vi "niRFSTS SG Set Waveform Names.vi"(0 "TSM Context in":T1, 5 "Waveform Names":string[](array[string]), 11 "error in (no error)":errorcluster) -> (4 "TSM Context out":T1, 15 "error out":errorcluster)   [LabVIEW 2014]
uses:
  <vilib>/NI_TestStand_SemiconductorModule/NI_TestStand_Semiconductor_Module.lvlibp/PinMap/General/SemiconductorModuleContext.ctl
  <vilib>/NI_TestStand_SemiconductorModule/NI_TestStand_Semiconductor_Module.lvlibp
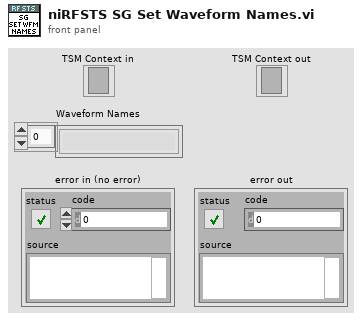
[diagram p1: front panel]
types:
  T1 = typedef "NI_TestStand_Semiconductor_Module.lvlibp/SemiconductorModuleContext.ctl" = refnum<k7>
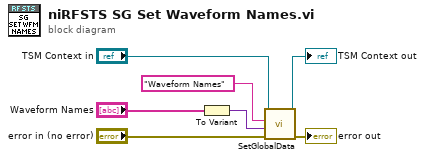
[diagram p0: block diagram]
diagram:
  n1 = To Variant(anything="Waveform Names") -> (Variant=w3:variant)
  n2 = call <vilib>:"SetGlobalData.vi"("error in (no error)"="error in (no error)", "Data"=w3, "Data Id"="Waveform Names", "Semiconductor Module Context"="TSM Context in") -> ("error out"=→"error out":errorcluster, "Semiconductor Module Context Out"=→"TSM Context out":T1)  [unwired: 5 in]
